vi "Extract image from stack.vi"(8 "error in (no error)":errorcluster, 11 "Selection":i32) -> (0 "error out":errorcluster, 1 "SNR":dbl, 2 "INtensity plot array":i16[][](array[numeric]), 3 "Refnum out":T1)   [LabVIEW 2020]
uses:
  <vilib>/vision/Image Controls.llb/IMAQ Image.ctl
  TypeDefs/data and image buffer fgv actions - measure tool.ctl
  <vilib>/Analysis/NI_AALBase.lvlib
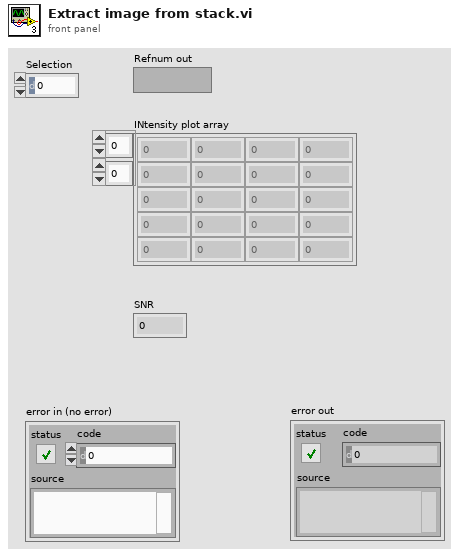
[diagram p1: front panel]
types:
  T1 = typedef "IMAQ Image.ctl" = refnum<image>
  T2 = typedef "data and image buffer fgv actions - measure tool.ctl" = enum16{"Initialise", "Load Data from file", "Add Image to buffer", "Read Image buffer", "Edit specific data", "Delete selected image", "Clear all images"}
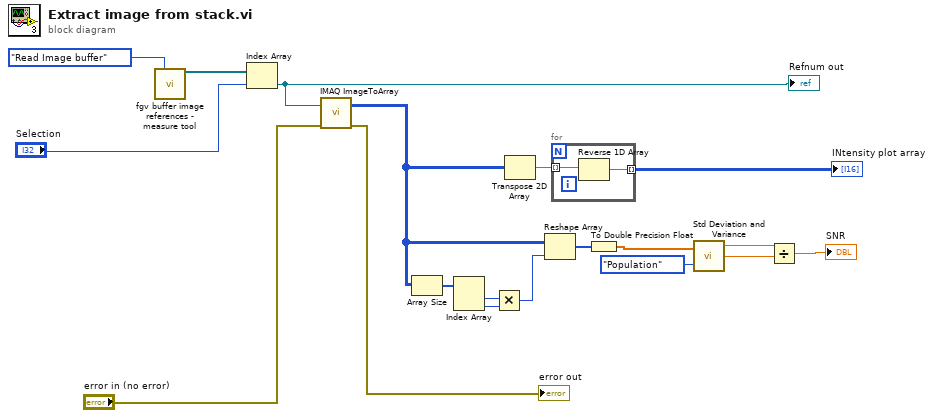
[diagram p0: block diagram]
diagram:
  n1 = call "fgv buffer image references - measure tool.vi"("Actions"=data_and_image_buffer_fgv_actions_-_measure_tool."Read Image buffer") -> ("Image Array"=w4:T1[])  [unwired: 8 in, 6 out]
  n2 = Index Array(array=w4, index="Selection") -> (element=w7:T1)
  "Refnum out" <- w7
  n3 = call "IMAQ ImageToArray"("error in (no error)"="error in (no error)", "Image"=w7) -> ("error out"=→"error out":errorcluster, "Image Pixels (I16)"=w9:i16[][])  [unwired: 2 in, 3 out]
  n4 = Array Size(array=w9) -> (size(s)=w10:i32[])
  n5 = Index Array(array=w10) -> (element #1=w12:i32, element #2=w11:i32)  [unwired: 2 in]
  n6 = Multiply(x=w12, y=w11) -> (x*y=w13:i32)
  n7 = Transpose 2D Array(2D array=w9) -> (transposed array=w6:i16[][])
  n8 = Reshape Array(w9, w13) -> (w14:i16[])
  n9 = for {
    tunnel: w6 -> [w21] mode=indexing
    tunnel: [w20] -> w5 mode=indexing
    n10 = Reverse 1D Array(array=w21) -> (reversed array=w20:i16[])
  }
  "INtensity plot array" <- w5
  n11 = To Double Precision Float(number=w14) -> (double precision float=w15:dbl[])
  n12 = call <vilib>:"Std Deviation and Variance.vi"("X"=w15, "Weighting (Sample)"=enum16{"Sample", "Population"}."Population") -> ("mean"=w17:dbl, "standard deviation"=w18:dbl)  [unwired: 1 out]
  n13 = Divide(x=w17, y=w18) -> (x/y=→"SNR":dbl)
